vi "AnalogIntegrator_NI5771_Resonance.vi"() -> ()   [LabVIEW 2012]
uses:
  <vilib>/Platform/TimedLoop/XDataNode/timing_clust.ctl
  <vilib>/Platform/TimedLoop/XDataNode/nitl_modes.ctl
  <vilib>/Platform/TimedLoop/XDataNode/wakeup.ctl
  <vilib>/rvi/FIFO/Fifo_Resource/nirvififoEmulationSetSize.vi
  <vilib>/rvi/DataTransferAndStorage/Container/Common/niFpgaContainerGetUniqueNameForEmu.vi
  <vilib>/rvi/eio/common/nirviEmuTemplateMethod_errors.vi
  <vilib>/rvi/Emulation/niFpgaSctlEmulationRegisterWithScheduler.vi
  <vilib>/rvi/errors/niFpgaSetErrorForExecOnDevCompSimple.vi
  <vilib>/rvi/eio/common/nirviEmuReportErrorAndStop.vi
  <vilib>/rvi/Emulation/niFpgaSctlEmulationFifoFullMgr.vi
  <vilib>/rvi/Emulation/niFpgaSctlEmulationResourceMgr.vi
  <vilib>/rvi/Emulation/niFpgaSctlEmulationScheduler.vi
  <vilib>/rvi/interface/RandomDataEmulation/nirviRandomDataFPGAFIFO.vi
  <vilib>/rvi/interface/RandomDataEmulation/niFpgaRandomDataHandleErrors.vi
  <vilib>/rvi/Emulation/niFpgaSctlEmulationGlobalWrite.vi
  <vilib>/Platform/TimedLoop/XDataNode/XDataNode.xnode
  <vilib>/rvi/DataTransferAndStorage/Container/XNode/niFpgaContainer.xnode
  <vilib>/rvi/FIFO/Fifo_Resource/nirvififoEmulationClear.vi
  <vilib>/eio/EIONode/EIONode.xnode
  <vilib>/rvi/FIFO/Fifo_Resource/nirvififoEmulationWrite.vi
  <vilib>/rvi/FIFO/Fifo_Resource/nirvififoEmulationRead.vi
  <vilib>/rvi/interface/RandomDataEmulation/nirviRandomDataFpgaReadWriteTemplate.vi
  <vilib>/Platform/TimedLoop/XDataNode/XDNodeRunTimeDep.lvlib
panel:
  out "Resonance Trigger":bool
  in  "Baselinex8 Ch2":u8
  in  "Baselinex8 Ch1":u8
  in  "Clear Interloop FIFO":bool
  out "InterloopFIFO Timeout":bool
  out "ToHostCh2FIFO Overflow":bool
  out "ToHostCh1FIFO Overflow":bool
  out "Pixel counter":u32
  in  "Wait for trigger":bool
  in  "Acquire":bool
  in  "Acquire continuously":bool=TRUE
  in  "Requested pixels":u32=100000
  out "InterloopFIFO Overflow":bool
  out "Acquiring":bool
  out "IO Module\\AI Over Range":bool
  in  "Samples per pixel":u32=10000 caption="Samples per pixel Acq"
  in  "Samples per line":u32=10000 caption="Samples per pixel Acq"
  in  "User Command Commit":bool
  in  "User Command":u8
  out "User Command Idle":bool
  out "User Command Status":u8
  in  "User Data 0":u16
  in  "User Data 1":u8
  out "PLL Locked":bool
  out "User Error":bool
  out "Configured?":bool
  # "5771 IO module configuration"
  # "Analog integrator"
  # "Acquisition control"
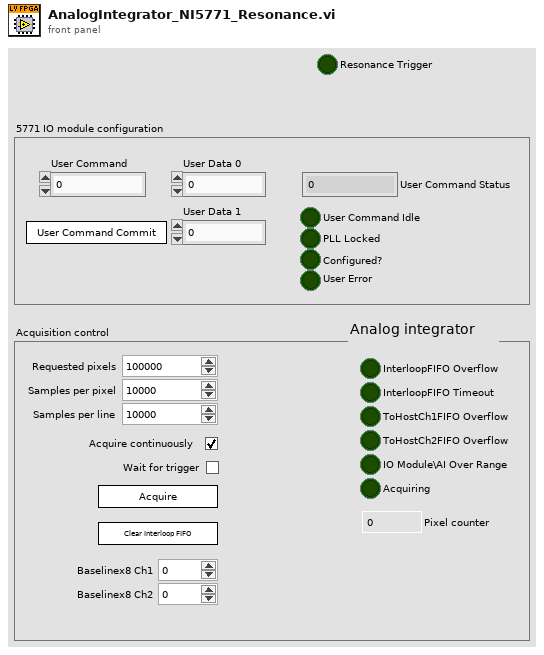
[diagram p1: front panel]
types:
  T1 = typedef "XDNodeRunTimeDep.lvlib/timing_clust.ctl" = cluster{"Expected End [f-1]":u64, "Actual End [f-1]":u64, "Finished Late? [f-1]":bool, "Expected End [i-1]":u64, "Actual End [i-1]":u64, "Finished Late? [i-1]":bool, "Expected Start [i]":u64, "Actual Start [i]":u64, "Expected Start [f]":u64, "Actual Start [f]":u64, "Source Name":string, "Structure Name":string, "Period":i64, "Deadline":i64, "Offset":i64, "Start":i64, "Priority":i32, "Timeout":i32, "Mode":T2, "Wakeup Reason":T3, "Error":errorcluster, "Source Type":string, "Secondary Source Type":string, "Global End Time":u64, "Global Start Time":u64, "Frame Duration":u64, "Iteration Duration":u64, "Assigned CPU":i32, "I/O Scan Engine Mode":u32}
  T2 = typedef "XDNodeRunTimeDep.lvlib/nitl_modes.ctl" = enum32{"No Change", "Process missed periods, maintain original phase", "Discard missed periods, maintain original phase", "Process missed periods, ignore original phase", "Discard missed periods, ignore original phase"}
  T3 = typedef "XDNodeRunTimeDep.lvlib/wakeup.ctl" = enum32{"Normal", "Aborted", "Asynchronous wakeup", "Timing source error", "Timed loop error", "Timeout"}
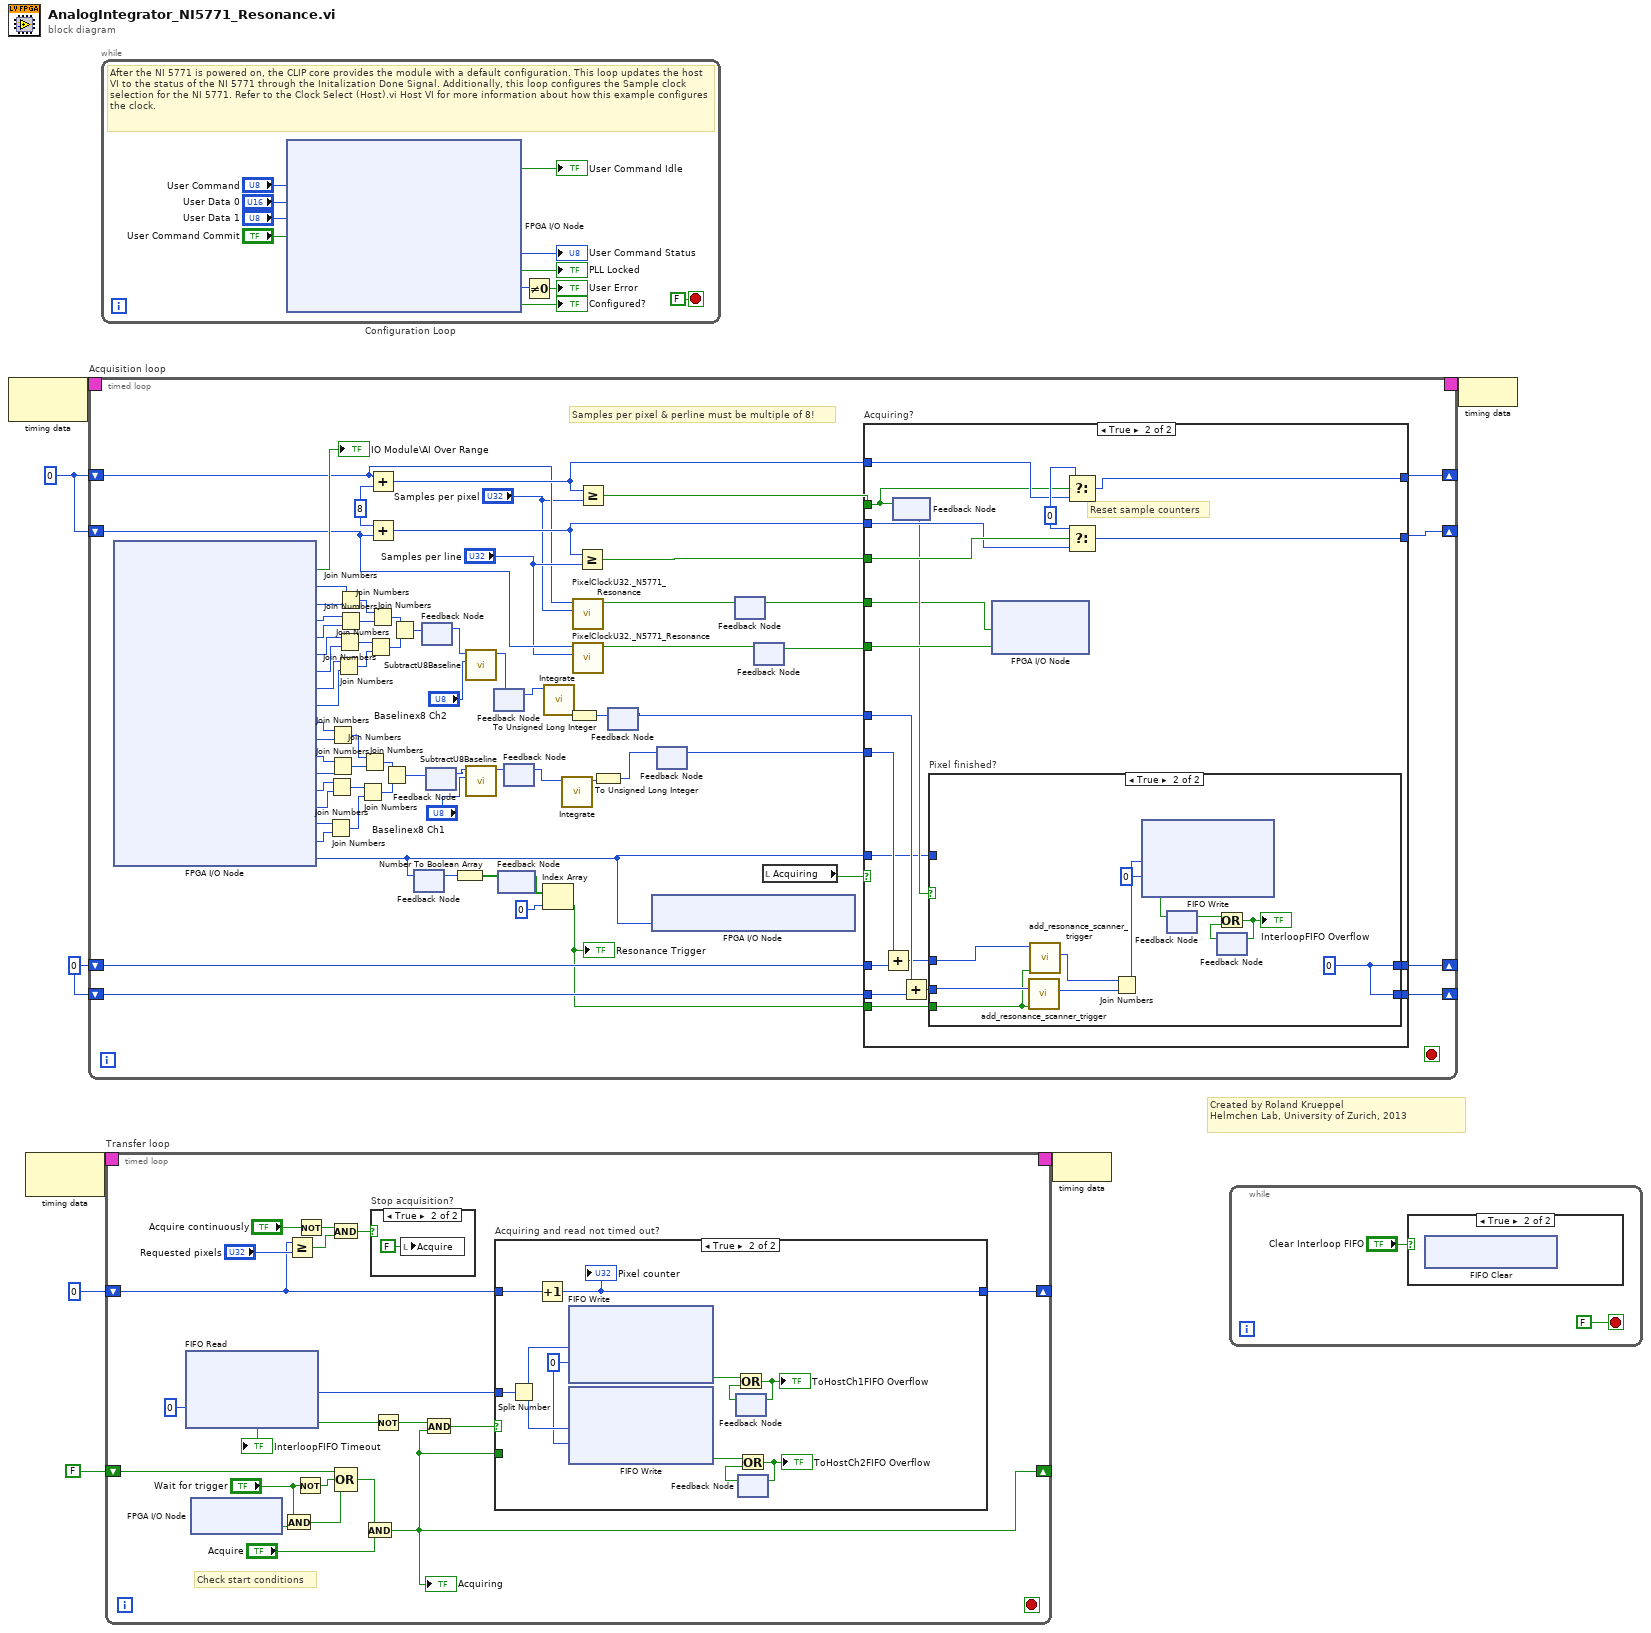
[diagram p0: block diagram]
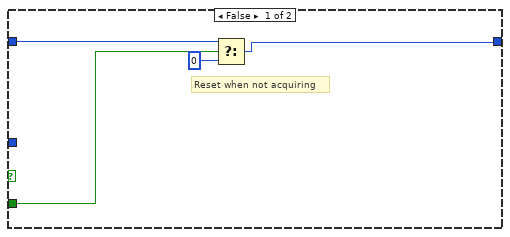
[diagram p4: hidden frame]
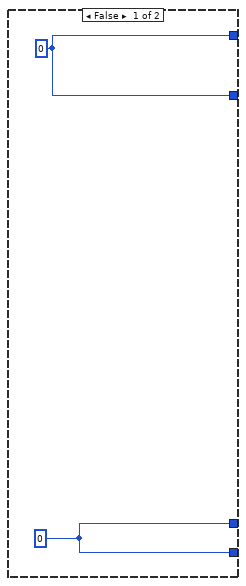
[diagram p5: hidden frame]
diagram:
  w5 = u32 0
  w6 = u32 0 ("t")
  # "Created by Roland Krueppel\nHelmchen Lab, University of Zurich, 2013"
  n1 = node-c288() -> (w8:T1)  [unwired: 1 in]
  n2 = node-c288() -> (w4:T1)  [unwired: 1 in]
  n3 = timed-loop "Acquisition loop" {
    timing: w8 -> [_]
    timing-out: [_] -> w7
    shift-right: [w78] -> _
    shift-left: w6 -> [w24]
    shift-right: [w79] -> _
    shift-left: w6 -> [w20]
    shift-right: [w74] -> _
    shift-left: w5 -> [w76]
    shift-right: [w73] -> _
    shift-left: w5 -> [w75]
    stop <- _ stop-if-true
    w72 = u32 8 ("y")
    # "Samples per pixel & perline must be multiple of 8!"
    n4 = xnode "FPGA I/O Node"() -> ("IO Module\\AI Over Range"=→"IO Module\\AI Over Range":bool, "IO Module\\AI 1 Data N-7"=w60:u8, "IO Module\\AI 1 Data N-6"=w59:u8, "IO Module\\AI 1 Data N-5"=w58:u8, "IO Module\\AI 1 Data N-4"=w57:u8, "IO Module\\AI 1 Data N-3"=w56:u8, "IO Module\\AI 1 Data N-2"=w55:u8, "IO Module\\AI 1 Data N-1"=w54:u8, "IO Module\\AI 1 Data N"=w53:u8, "IO Module\\AI 0 Data N-7"=w37:u8, "IO Module\\AI 0 Data N-6"=w36:u8, "IO Module\\AI 0 Data N-5"=w35:u8, "IO Module\\AI 0 Data N-4"=w34:u8, "IO Module\\AI 0 Data N-3"=w33:u8, "IO Module\\AI 0 Data N-2"=w32:u8, "IO Module\\AI 0 Data N-1"=w31:u8, "IO Module\\AI 0 Data N"=w38:u8, "IO Module\\DIO Port 0 Rd Data"=w62:u8)  [unwired: 18 in, 18 out]
    n5 = Join Numbers(hi=w31, lo=w38) -> ((hi.lo)=w42:u16)
    n6 = Join Numbers(hi=w33, lo=w32) -> ((hi.lo)=w43:u16)
    n7 = Join Numbers(hi=w37, lo=w36) -> ((hi.lo)=w45:u16)
    n8 = Join Numbers(hi=w35, lo=w34) -> ((hi.lo)=w44:u16)
    n9 = Join Numbers(hi=w54, lo=w53) -> ((hi.lo)=w49:u16)
    n10 = Join Numbers(hi=w56, lo=w55) -> ((hi.lo)=w50:u16)
    n11 = Join Numbers(hi=w60, lo=w59) -> ((hi.lo)=w52:u16)
    n12 = Join Numbers(hi=w58, lo=w57) -> ((hi.lo)=w51:u16)
    n13 = Join Numbers(hi=w43, lo=w42) -> ((hi.lo)=w40:u32)
    n14 = Join Numbers(hi=w45, lo=w44) -> ((hi.lo)=w41:u32)
    n15 = Join Numbers(hi=w50, lo=w49) -> ((hi.lo)=w47:u32)
    n16 = Add(x=w20, y=w72) -> (x+y=w27:u32)
    n17 = Add(x=w72, y=w24) -> (x+y=w29:u32)
    n18 = Join Numbers(hi=w52, lo=w51) -> ((hi.lo)=w48:u32)
    n19 = Join Numbers(hi=w41, lo=w40) -> ((hi.lo)=w39:u64)
    n20 = Join Numbers(hi=w48, lo=w47) -> ((hi.lo)=w46:u64)
    n21 = feedback #1() -> (w61:u8)  [unwired: 1 in]
    n22 = feedback-in #1(w62) -> ()
    n23 = feedback #2() -> (w16:u64)  [unwired: 1 in]
    n24 = feedback-in #2(w46) -> ()
    n25 = feedback #3() -> (w12:u64)  [unwired: 1 in]
    n26 = feedback-in #3(w39) -> ()
    n27 = Number To Boolean Array(number=w61) -> (Boolean array=w65:bool[])
    n28 = call "SubtractU8Baseline.vi"("Baseline U8"="Baselinex8 Ch2", "New samples in"=w16) -> ("New samples out"=w15:u64)  [unwired: 9 in]
    n29 = call "SubtractU8Baseline.vi"("Baseline U8"="Baselinex8 Ch1", "New samples in"=w12) -> ("New samples out"=w11:u64)  [unwired: 9 in]
    n30 = feedback #4() -> (w18:u64)  [unwired: 1 in]
    n31 = feedback-in #4(w15) -> ()
    n32 = feedback #5() -> (w66:bool[])  [unwired: 1 in]
    n33 = feedback-in #5(w65) -> ()
    n34 = feedback #6() -> (w10:u64)  [unwired: 1 in]
    n35 = feedback-in #6(w11) -> ()
    n36 = Index Array(array=w66, index=0) -> (element=w63:bool)
    "Resonance Trigger" <- w63
    n37 = call "Integrate.vi"("New samples in"=w18) -> ("Sum out"=w17:u16)  [unwired: 9 in, 1 out]
    n38 = call "Integrate.vi"("New samples in"=w10) -> ("Sum out"=w9:u16)  [unwired: 9 in, 1 out]
    n39 = To Unsigned Long Integer(number=w17) -> (unsigned 32bit integer=w70:u32)
    n40 = call "PixelClockU32._N5771_Resonance.vi"("Samples per pixel"="Samples per pixel", "Sample counter"=w20) -> ("Pixel clock"=w21:bool)  [unwired: 9 in]
    n41 = call "PixelClockU32._N5771_Resonance.vi"("Samples per pixel"="Samples per line", "Sample counter"=w24) -> ("Pixel clock"=w22:bool)  [unwired: 9 in]
    n42 = Greater Or Equal?(x=w29, y="Samples per line") -> (x >= y?=w30:bool)
    n43 = Greater Or Equal?(x=w27, y="Samples per pixel") -> (x >= y?=w28:bool)
    n44 = To Unsigned Long Integer(number=w9) -> (unsigned 32bit integer=w68:u32)
    n45 = feedback #7() -> (w69:u32)  [unwired: 1 in]
    n46 = feedback-in #7(w70) -> ()
    n47 = xnode "FPGA I/O Node"("IO Module\\DIO Port 1 Wr Data"=w62) -> ()  [unwired: 1 in, 1 out]
    n48 = feedback #8() -> (w67:u32)  [unwired: 1 in]
    n49 = feedback-in #8(w68) -> ()
    n50 = feedback #9() -> (w25:bool)  [unwired: 1 in]
    n51 = feedback-in #9(w21) -> ()
    n52 = feedback #10() -> (w26:bool)  [unwired: 1 in]
    n53 = feedback-in #10(w22) -> ()
    n54 = local read "Acquiring"() -> (w77:bool)
    n55 = case "Acquiring?" shown="True" w77 {
      tunnel: [w81 w100] -> w79
      tunnel: [w81 w99] -> w78
      tunnel: w67 -> [_ w98]
      tunnel: w76 -> [_ w87]
      tunnel: w75 -> [_ w97]
      tunnel: w69 -> [_ w96]
      tunnel: [w80 w95] -> w74
      tunnel: [w80 w94] -> w73
      tunnel: w28 -> [_ w89]
      tunnel: w30 -> [_ w93]
      tunnel: w27 -> [_ w92]
      tunnel: w29 -> [_ w91]
      tunnel: w25 -> [_ w82]
      tunnel: w26 -> [_ w90]
      tunnel: w62 -> [_ w84]
      tunnel: w63 -> [_ w83]
      frame False {
        w80 = u32 0
        w81 = u16 0 ("t")
      }
      frame True {
        w101 = u32 0 ("t")
        # "Reset sample counters"
        n56 = Add(x=w98, y=w87) -> (x+y=w86:u32)
        n57 = feedback #11() -> (w88:bool)  [unwired: 1 in]
        n58 = feedback-in #11(w89) -> ()
        n59 = Add(x=w96, y=w97) -> (x+y=w85:u32)
        n60 = case "Pixel finished?" shown="True" w88 {
          tunnel: w85 -> [w103 w106]
          tunnel: w86 -> [w102 w105]
          tunnel: [w102 w111] -> w95
          tunnel: [w103 w111] -> w94
          tunnel: w84 -> [_ _]
          tunnel: w83 -> [_ w104]
          frame False {
          }
          frame True {
            w111 = u32 0
            n61 = call "add_resonance_scanner_trigger.vi"("Trigger"=w104, "Input"=w106) -> ("Output"=w107:u32)  [unwired: 9 in]
            n62 = call "add_resonance_scanner_trigger.vi"("Trigger"=w104, "Input"=w105) -> ("Output"=w108:u32)  [unwired: 9 in]
            n63 = Join Numbers(hi=w108, lo=w107) -> ((hi.lo)=w115:u64)
            n64 = xnode ("FIFO Write")("Element"=w115, "Timeout"=0) -> ("Timed Out?"=w109:bool)  [unwired: 1 in, 1 out]
            n65 = feedback-in #12(w109) -> ()
            n66 = feedback #12() -> (w110:bool)  [unwired: 1 in]
            n67 = feedback #13() -> (w112:bool)  [unwired: 1 in]
            n68 = Or(x=w110, y=w112) -> (x .or. y?=w113:bool)
            "InterloopFIFO Overflow" <- w113
            n69 = feedback-in #13(w113) -> ()
          }
        }
        n70 = xnode "FPGA I/O Node"("PixelClock"=w82, "LineClock"=w90) -> ()  [unwired: 2 in, 2 out]
        n71 = Select(t=w101, s=w89, f=w92) -> (s? t:f=w100:u32)
        n72 = Select(t=w101, s=w93, f=w91) -> (s? t:f=w99:u32)
      }
    }
  }
  n73 = while "Configuration Loop" {
    stop <- FALSE stop-if-true
    # "After the NI 5771 is powered on, the CLIP core provides the module with a default configuration. This loop updates the host VI to the status of the NI 5771 through the Initalization Done Signal. Additionally, this loop configures the Sample clock selection for the NI 5771. Refer to the Clock Select (Host).vi Host VI for more information about how this example configures the clock."
    n74 = xnode "FPGA I/O Node"("IO Module\\User Command"="User Command", "IO Module\\User Data 0"="User Data 0", "IO Module\\User Data 1"="User Data 1", "IO Module\\User Command Commit"="User Command Commit") -> ("IO Module\\User Command Idle"=→"User Command Idle":bool, "IO Module\\User Command Status"=→"User Command Status":u8, "IO Module\\PLL Locked"=→"PLL Locked":bool, "IO Module\\User Error"=w121:u8, "IO Module\\Initialization Done"=→"Configured?":bool)  [unwired: 9 in, 9 out]
    n75 = Not Equal To 0?(x=w121) -> (x != 0?=→"User Error":bool)
  }
  n76 = timed-loop "Transfer loop" {
    timing: w4 -> [_]
    timing-out: [_] -> w3
    shift-right: [w131] -> _
    shift-left: u32 0 -> [w132]
    shift-right: [w130] -> _
    shift-left: FALSE -> [w138]
    stop <- _ stop-if-true
    # "Check start conditions"
    n77 = xnode ("FIFO Read")("Timeout"=0) -> ("Element"=w133:u64, "Timed Out?"=w137:bool)  [unwired: 1 in, 1 out]
    "InterloopFIFO Timeout" <- w137
    n78 = xnode "FPGA I/O Node"() -> ("TriggerIn"=w143:bool)  [unwired: 1 in, 1 out]
    n79 = And(x="Wait for trigger", y=w143) -> (x .and. y?=w140:bool)
    n80 = Greater Or Equal?(x=w132, y="Requested pixels") -> (x >= y?=w145:bool)
    n81 = Not(x="Wait for trigger") -> (.not. x?=w141:bool)
    n82 = Not(x="Acquire continuously") -> (.not. x?=w146:bool)
    n83 = And(x=w146, y=w145) -> (x .and. y?=w135:bool)
    n84 = Compound Arithmetic op=OR(w138, w141, w140) -> (w139:bool)
    n85 = And(x=w139, y="Acquire") -> (x .and. y?=w130:bool)
    "Acquiring" <- w130
    n86 = case "Stop acquisition?" shown="True" w135 {
      frame False {
      }
      frame True {
        n87 = local write "Acquire"(FALSE ("Acquire")) -> ()
      }
    }
    n88 = Not(x=w137) -> (.not. x?=w136:bool)
    n89 = And(x=w136, y=w130) -> (x .and. y?=w134:bool)
    n90 = case "Acquiring and read not timed out?" shown="True" w134 {
      tunnel: w133 -> [_ w165]
      tunnel: w132 -> [w152 w161]
      tunnel: [w151 w160] -> w131
      tunnel: w130 -> [w153 _]
      frame False {
        # "Reset when not acquiring"
        n91 = Select(t=w152, s=w153, f=u32 0) -> (s? t:f=w151:u32)
      }
      frame True {
        w162 = 0 ("Timeout")
        n92 = Split Number(x=w165) -> (hi(x)=w164:u32, lo(x)=w163:u32)
        n93 = Increment(x=w161) -> (x+1=w160:u32)
        "Pixel counter" <- w160
        n94 = xnode ("FIFO Write")("Element"=w164, "Timeout"=w162) -> ("Timed Out?"=w158:bool)  [unwired: 1 in, 1 out]
        n95 = xnode ("FIFO Write")("Element"=w163, "Timeout"=w162) -> ("Timed Out?"=w155:bool)  [unwired: 1 in, 1 out]
        n96 = feedback #14() -> (w157:bool)  [unwired: 1 in]
        n97 = Or(x=w158, y=w157) -> (x .or. y?=w159:bool)
        "ToHostCh1FIFO Overflow" <- w159
        n98 = feedback-in #14(w159) -> ()
        n99 = feedback #15() -> (w154:bool)  [unwired: 1 in]
        n100 = Or(x=w155, y=w154) -> (x .or. y?=w156:bool)
        "ToHostCh2FIFO Overflow" <- w156
        n101 = feedback-in #15(w156) -> ()
      }
    }
  }
  n102 = node-c288(w3) -> ()
  n103 = while {
    stop <- FALSE stop-if-true
    n104 = case shown="True" "Clear Interloop FIFO" {
      frame False {
      }
      frame True {
        n105 = xnode ("FIFO Clear")() -> ()  [unwired: 1 in, 1 out]
      }
    }
  }
  n106 = node-c288(w7) -> ()
